vi "CoordinateConvert_CartesianToArm_Arrays.vi"(1 "XYPoints":T1[](array[typedef])) -> (0 "ArmCoordinates":T2[](array[typedef]))   [LabVIEW 2018]
uses:
  TypeDefs/ArmCoordinate.ctl
  ArgosLib/Path Planning/TypeDefs/Point2D.ctl
  ArgosLib/ArgosLib.lvlib
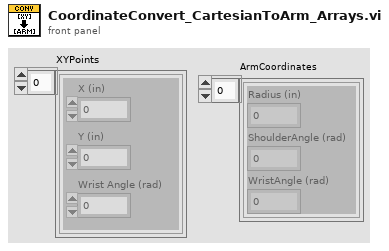
[diagram p1: front panel]
types:
  T1 = typedef "ArgosLib.lvlib/Point2D.ctl" = cluster{"X (in)":dbl, "Y (in)":dbl, "Wrist Angle (rad)":dbl}
  T2 = typedef "ArmCoordinate.ctl" = cluster{"Radius (in)":dbl, "ShoulderAngle (rad)":dbl, "WristAngle (rad)":dbl}
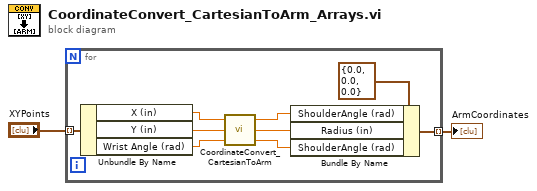
[diagram p0: block diagram]
diagram:
  n1 = for {
    tunnel: "XYPoints" -> [w11] mode=indexing
    tunnel: [w7] -> w1 mode=indexing
    n2 = Unbundle By Name(w11) -> ("X (in)"=w10:dbl, "Y (in)"=w6:dbl, "Wrist Angle (rad)"=w5:dbl)
    n3 = call "CoordinateConvert_CartesianToArm.vi"("Wrist (rad)"=w5, "Y (in)"=w6, "X (in)"=w10) -> ("Wrist Angle (rad)"=w4:dbl, "Radius (in)"=w3:dbl, "Shoulder Angle (rad)"=w9:dbl)
    n4 = Bundle By Name(cluster=T2 {"Radius (in)"=0.0, "ShoulderAngle (rad)"=0.0, "WristAngle (rad)"=0.0} ("Point"), "ShoulderAngle (rad)"=w9, "Radius (in)"=w3, "ShoulderAngle (rad)"=w4) -> (w7:T2)
  }
  "ArmCoordinates" <- w1
